vi "getSenMfromFile.vi"(8 "error in (no error)":errorcluster, 9 "Sensitivity Matrix Shape":T1={"Num of Field"=35, "Num of Zk"=19, "Num of DOF"=50}, 10 "Path":path=path "/home/ttsai/Documents/stash/ts_tcs_ofc/configData/lsst/senM_35_19_50.txt", 11 "MatOper in":refnum<class "MatOper.lvclass">) -> (0 "error out":errorcluster, 2 "Sensitivity Matrix":dbl[][][](array[numeric]), 3 "MatOper out":refnum<class "MatOper.lvclass">)   [LabVIEW 2016, in "MatOper.lvclass"]
doc: "Get the sensitivity matrix M from txt file."
uses:
  MatOper.lvclass
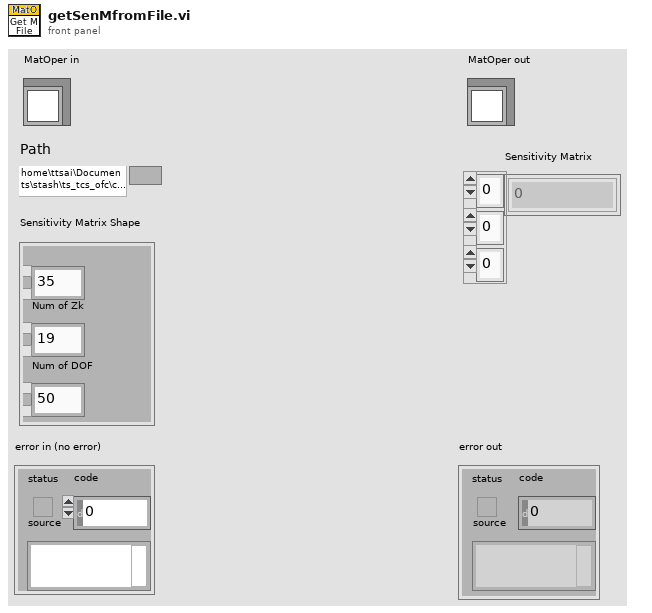
[diagram p1: front panel]
types:
  T1 = cluster{"Num of Field":i32, "Num of Zk":i32, "Num of DOF":i32}
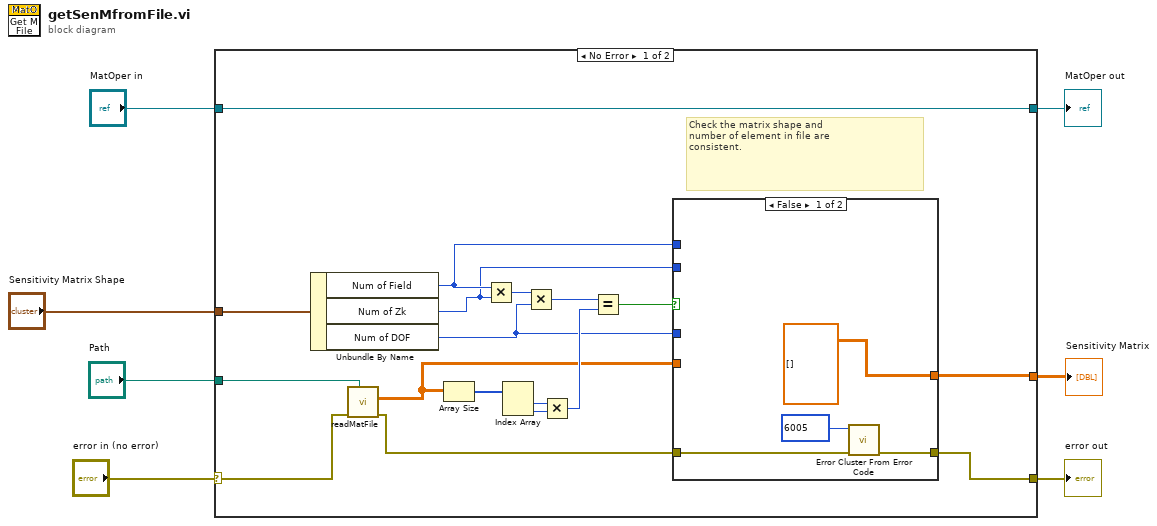
[diagram p0: block diagram]
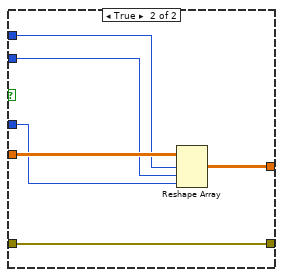
[diagram p2: hidden frame]
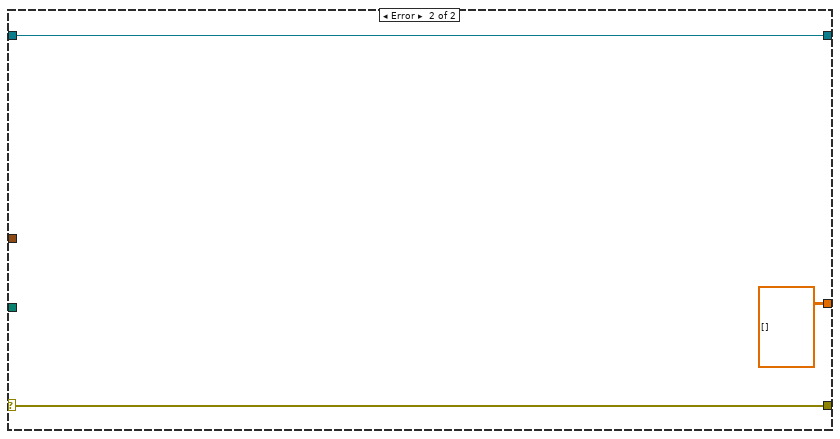
[diagram p3: hidden frame]
diagram:
  n1 = case shown="No Error" "error in (no error)" {
    selector: "error in (no error)" -> [w11 w38]
    tunnel: [w12 w38] -> w6
    tunnel: [w25 w37] -> w4
    tunnel: "MatOper in" -> [w25 w37]
    tunnel: "Sensitivity Matrix Shape" -> [w10 _]
    tunnel: "Path" -> [w8 _]
    tunnel: [w9 dbl[][][] [] ("Matrix")] -> w1
    frame No Error {
      # "Check the matrix shape and \nnumber of element in file are\nconsistent."
      n2 = Unbundle By Name(w10) -> ("Num of Field"=w15:i32, "Num of Zk"=w14:i32, "Num of DOF"=w13:i32)
      n3 = call "readMatFile.vi"("Path"=w8, "error in (no error)"=w11) -> ("error out"=w17:errorcluster, "Matrix"=w16:dbl[][])  [unwired: 7 in, 1 out]
      n4 = Array Size(array=w16) -> (size(s)=w23:i32[])
      n5 = Multiply(x=w15, y=w14) -> (x*y=w24:i32)
      n6 = Index Array(array=w23) -> (element #1=w22:i32, element #2=w21:i32)  [unwired: 2 in]
      n7 = Multiply(x=w24, y=w13) -> (x*y=w19:i32)
      n8 = Multiply(x=w22, y=w21) -> (x*y=w20:i32)
      n9 = Equal?(x=w19, y=w20) -> (x = y?=w18:bool)
      n10 = case shown="False" w18 {
        tunnel: w17 -> [w28 w30]
        tunnel: [w27 w30] -> w12
        tunnel: w16 -> [_ w35]
        tunnel: w15 -> [_ w34]
        tunnel: w14 -> [_ w33]
        tunnel: w13 -> [_ w32]
        tunnel: [dbl[][][] [] ("Matrix") w31] -> w9
        frame False {
          n11 = call <vilib>:"Error Cluster From Error Code.vi"("error in (no error)"=w28, "error code (0)"=6005 ("code")) -> ("error out"=w27:errorcluster)  [unwired: 7 in]
        }
        frame True {
          n12 = Reshape Array(w35, w34, w33, w32) -> (w31:dbl[][][])
        }
      }
    }
    frame Error {
    }
  }
  "error out" <- w6
  "MatOper out" <- w4
  "Sensitivity Matrix" <- w1
